vi "trace.payload_received.vi"(10 "Response":string="<empty string>", 11 "Path":string) -> ()   [LabVIEW 2020, in "Nominal Client.lvclass"]
uses:
  Nominal Client.lvclass
  <vilib>/Utility/libraryn.llb/Get File Extension.vi
  Nominal Client.lvclass/Nominal Client.ctl
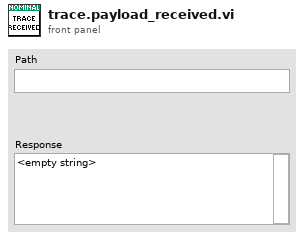
[diagram p1: front panel]
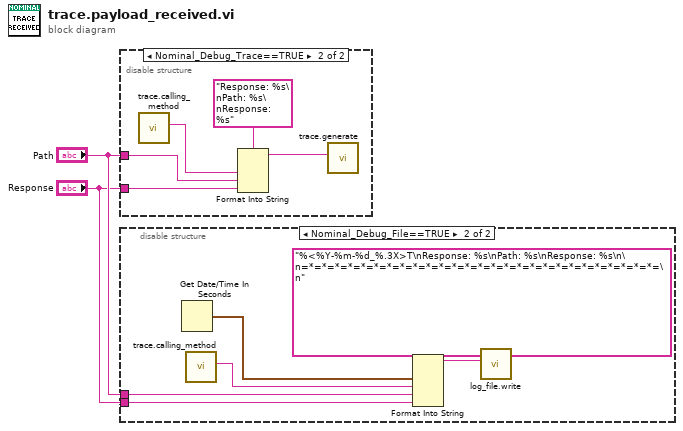
[diagram p0: block diagram]
diagram:
  n1 = disable-structure shown="Nominal_Debug_Trace==TRUE" {
    disable-tunnel: "Response" -> [_ w6]
    disable-tunnel: "Path" -> [_ w5]
    frame condition #0 {
    }
    frame condition #1 (active) {
      n2 = call "trace.calling_method.vi"() -> ("Calling Method Name"=w3:string)  [unwired: 11 in]
      n3 = Format Into String(format string="Response: %s\nPath: %s\nResponse: %s", w3, w5, w6) -> (resulting string=w7:string)  [unwired: 2 in, 1 out]
      n4 = call "trace.generate.vi"("trace string"=w7) -> ()  [unwired: 11 in]
    }
  }
  n5 = disable-structure shown="Nominal_Debug_File==TRUE" {
    disable-tunnel: "Response" -> [_ w13]
    disable-tunnel: "Path" -> [_ w12]
    frame condition #0 {
    }
    frame condition #1 (active) {
      n6 = Get Date/Time In Seconds() -> (seconds since 1Jan1904=w8:timestamp)
      n7 = call "trace.calling_method.vi"() -> ("Calling Method Name"=w10:string)  [unwired: 11 in]
      n8 = Format Into String(format string="%<%Y-%m-%d_%.3X>T\nResponse: %s\nPath: %s\nResponse: %s\n\n=*=*=*=*=*=*=*=*=*=*=*=*=*=*=*=*=*=*=*=*=*=*=*=*=*=*=*=\n", w8, w10, w12, w13) -> (resulting string=w9:string)  [unwired: 2 in, 1 out]
      n9 = call "log_file.write.vi"("trace string"=w9) -> ()  [unwired: 11 in]
    }
  }
